vi "Send TCP Command.vi"(7 "Action":T1, 8 "error in (no error)":errorcluster, 10 "Custom Message":string, 11 "Telnet V2 in":refnum<class "Telnet V2.lvclass">) -> (0 "error out":errorcluster, 3 "Telnet V2 out":refnum<class "Telnet V2.lvclass">)   [LabVIEW 2018, in "Telnet V2.lvlib" / "Telnet V2.lvclass"]
uses:
  Telnet V2.lvclass
  PPLs/LiDAR/Parent/LiDAR.lvlibp/Controls/enm_Actions_for_LiDAR.ctl
  Controls/enum_Telnet_Actions.ctl
  PPLs/LiDAR/Parent/LiDAR.lvlibp/LiDAR.lvclass
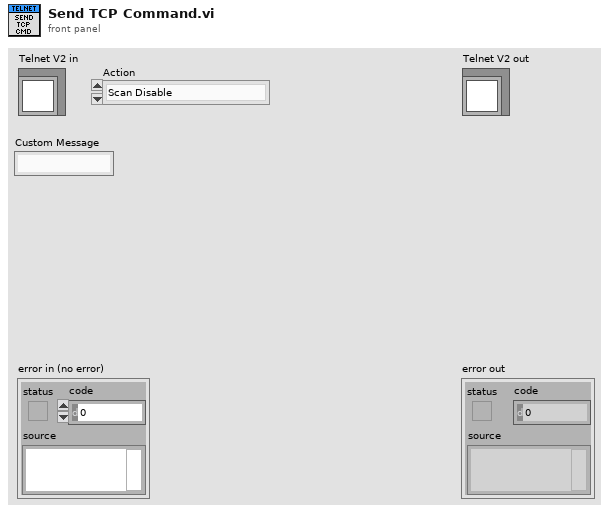
[diagram p1: front panel]
types:
  T1 = typedef "LiDAR.lvlibp/LiDAR.lvclass/enm_Actions_for_LiDAR.ctl" = enum16{"Scan Disable", "Scan Enable", "Standby", "Active", "Change EL Scan", "Change AZ Scan", "Change Algo", "Custom"}
  T2 = typedef "Telnet V2.lvlib/Telnet V2.lvclass/enum_Telnet_Actions.ctl" = enum16{"Scan Enable", "Scan Disable", "Active", "Standby", "Change EL Scan", "Change AZ Scan", "Set Data Algo", "Debug System", "Debug Laser", "Exit"}
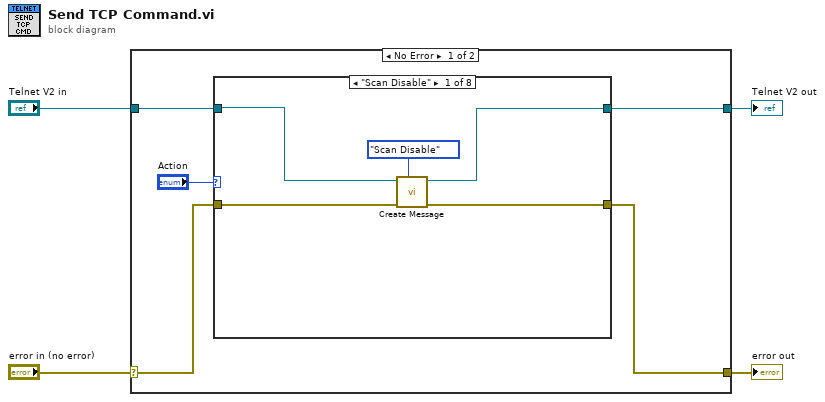
[diagram p0: block diagram]
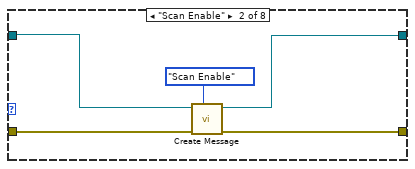
[diagram p2: hidden frame]
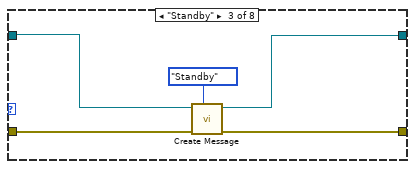
[diagram p3: hidden frame]
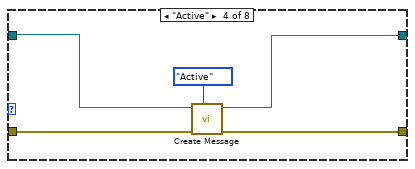
[diagram p4: hidden frame]
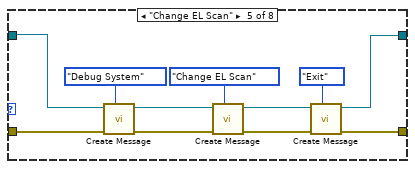
[diagram p5: hidden frame]
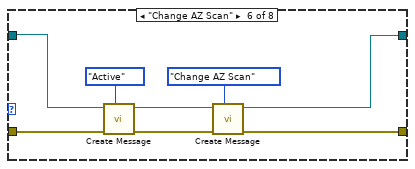
[diagram p6: hidden frame]
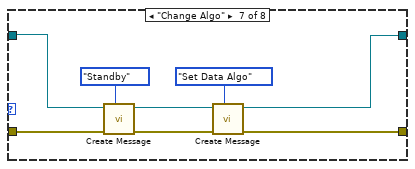
[diagram p7: hidden frame]
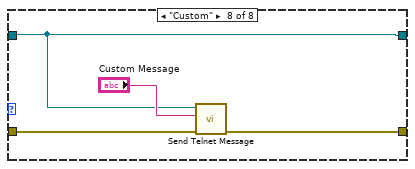
[diagram p8: hidden frame]
diagram:
  n1 = case shown="No Error" "error in (no error)" {
    selector: "error in (no error)" -> [w7 w62]
    tunnel: [w6 w62] -> w3
    tunnel: [w5 w61] -> w1
    tunnel: "Telnet V2 in" -> [w8 w61]
    frame No Error {
      n2 = case shown="\"Scan Disable\"" "Action" {
        tunnel: w8 -> [w13 w18 w23 w28 w39 w47 w55 w57]
        tunnel: w7 -> [w11 w16 w20 w26 w32 w43 w51 w59]
        tunnel: [w10 w15 w21 w25 w31 w41 w49 w58] -> w6
        tunnel: [w12 w17 w22 w27 w30 w42 w50 w57] -> w5
        frame "Scan Disable" {
          n3 = call "Create Message.vi"("Action"=enum_Telnet_Actions."Scan Disable", "error in (no error)"=w11, "Telnet V2 in"=w13) -> ("error out"=w10:errorcluster, "Telnet V2 Out"=w12:refnum<class "Telnet V2.lvclass">)  [unwired: 7 in]
        }
        frame "Scan Enable" {
          n4 = call "Create Message.vi"("Action"=enum_Telnet_Actions."Scan Enable", "error in (no error)"=w16, "Telnet V2 in"=w18) -> ("error out"=w15:errorcluster, "Telnet V2 Out"=w17:refnum<class "Telnet V2.lvclass">)  [unwired: 7 in]
        }
        frame "Standby" {
          n5 = call "Create Message.vi"("Action"=enum_Telnet_Actions."Standby", "error in (no error)"=w20, "Telnet V2 in"=w23) -> ("error out"=w21:errorcluster, "Telnet V2 Out"=w22:refnum<class "Telnet V2.lvclass">)  [unwired: 7 in]
        }
        frame "Active" {
          n6 = call "Create Message.vi"("Action"=enum_Telnet_Actions."Active", "error in (no error)"=w26, "Telnet V2 in"=w28) -> ("error out"=w25:errorcluster, "Telnet V2 Out"=w27:refnum<class "Telnet V2.lvclass">)  [unwired: 7 in]
        }
        frame "Change EL Scan" {
          n7 = call "Create Message.vi"("Action"=enum_Telnet_Actions."Debug System", "error in (no error)"=w32, "Telnet V2 in"=w39) -> ("error out"=w37:errorcluster, "Telnet V2 Out"=w38:refnum<class "Telnet V2.lvclass">)  [unwired: 7 in]
          n8 = call "Create Message.vi"("Action"=enum_Telnet_Actions."Change EL Scan", "error in (no error)"=w37, "Telnet V2 in"=w38) -> ("error out"=w33:errorcluster, "Telnet V2 Out"=w34:refnum<class "Telnet V2.lvclass">)  [unwired: 7 in]
          n9 = call "Create Message.vi"("Action"=enum_Telnet_Actions."Exit", "error in (no error)"=w33, "Telnet V2 in"=w34) -> ("error out"=w31:errorcluster, "Telnet V2 Out"=w30:refnum<class "Telnet V2.lvclass">)  [unwired: 7 in]
        }
        frame "Change AZ Scan" {
          n10 = call "Create Message.vi"("Action"=enum_Telnet_Actions."Active", "error in (no error)"=w43, "Telnet V2 in"=w47) -> ("error out"=w45:errorcluster, "Telnet V2 Out"=w46:refnum<class "Telnet V2.lvclass">)  [unwired: 7 in]
          n11 = call "Create Message.vi"("Action"=enum_Telnet_Actions."Change AZ Scan", "error in (no error)"=w45, "Telnet V2 in"=w46) -> ("error out"=w41:errorcluster, "Telnet V2 Out"=w42:refnum<class "Telnet V2.lvclass">)  [unwired: 7 in]
        }
        frame "Change Algo" {
          n12 = call "Create Message.vi"("Action"=enum_Telnet_Actions."Standby", "error in (no error)"=w51, "Telnet V2 in"=w55) -> ("error out"=w53:errorcluster, "Telnet V2 Out"=w54:refnum<class "Telnet V2.lvclass">)  [unwired: 7 in]
          n13 = call "Create Message.vi"("Action"=enum_Telnet_Actions."Set Data Algo", "error in (no error)"=w53, "Telnet V2 in"=w54) -> ("error out"=w49:errorcluster, "Telnet V2 Out"=w50:refnum<class "Telnet V2.lvclass">)  [unwired: 7 in]
        }
        frame "Custom" {
          n14 = call "Send Telnet Message.vi"("error in"=w59, "Message In"="Custom Message", "Telnet V2 in"=w57) -> ("error out"=w58:errorcluster)  [unwired: 8 in]
        }
      }
    }
    frame Error {
    }
  }
  "error out" <- w3
  "Telnet V2 out" <- w1
